vi "UHR-Fleezers Control (host) - 10.7.vi"() -> ()   [LabVIEW 2011] (continued)
  out "All Signals":waveform(dbl)[](graph)=[{"t0"=timestamp(6362.100000002397 s since 1904-01-01), "dt"=0.15, "Y"=[0.0, 0.0], "attributes"=variant("NI_ChannelName"=variant(string "APD 1"))}, {"t0"=timestamp(6362.100000002397 s since 1904-01-01), "dt"=0.15, "Y"=[0.0, 0.0], "attributes"=variant("NI_ChannelName"=variant(string "APD 2"))}, {"t0"=timestamp(6362.100000002397 s since 1904-01-01), "dt"=0.15, "Y"=[-0.08338581231742673, -0.0833608577290399], "attributes"=variant("NI_ChannelName"=variant(string "T1 Y"))}, {"t0"=timestamp(6362.100000002397 s since 1904-01-01), "dt"=0.15, "Y"=[-0.020466167643691944, -0.020695046740946327], "attributes"=variant("NI_ChannelName"=variant(string "T1 X"))}, {"t0"=timestamp(6362.100000002397 s since 1904-01-01), "dt"=0.15, "Y"=[0.05484865871150737, 0.05486028626361772], "attributes"=variant("NI_ChannelName"=variant(string "T1 Sum"))}, {"t0"=timestamp(6362.100000002397 s since 1904-01-01), "dt"=0.15, "Y"=[-0.08425842785872134, -0.08429414541514367], "attributes"=variant("NI_ChannelName"=variant(string "T2 Y"))}, {"t0"=timestamp(6362.100000002397 s since 1904-01-01), "dt"=0.15, "Y"=[-0.021052391190805018, -0.02125588256402392], "attributes"=variant("NI_ChannelName"=variant(string "T2 X"))}, {"t0"=timestamp(6362.100000002397 s since 1904-01-01), "dt"=0.15, "Y"=[0.054857295449689085, 0.05486660359507926], "attributes"=variant("NI_ChannelName"=variant(string "T2 Sum"))}, {"t0"=timestamp(6362.100000002397 s since 1904-01-01), "dt"=0.15, "Y"=[0.0185221741108709, 0.01777471038140605], "attributes"=variant("NI_ChannelName"=variant(string "T1 FB X"))}, {"t0"=timestamp(6362.100000002397 s since 1904-01-01), "dt"=0.15, "Y"=[0.007208807641834616, 0.007202642902920465], "attributes"=variant("NI_ChannelName"=variant(string "T1 FB Sum"))}, {"t0"=timestamp(6362.100000002397 s since 1904-01-01), "dt"=0.15, "Y"=[0.01339629623834087, 0.012486021324128876], "attributes"=variant("NI_ChannelName"=variant(string "T2 FB X"))}, {"t0"=timestamp(6362.100000002397 s since 1904-01-01), "dt"=0.15, "Y"=[0.007181218909268317, 0.007177312540055389], "attributes"=variant("NI_ChannelName"=variant(string "T2 FB Sum"))}, {"t0"=timestamp(6362.100000002397 s since 1904-01-01), "dt"=0.15, "Y"=[3.0154429223543846, 3.015887654048213], "attributes"=variant("NI_ChannelName"=variant(string "PSD Y"))}, {"t0"=timestamp(6362.100000002397 s since 1904-01-01), "dt"=0.15, "Y"=[0.1874808590976985, 0.18613934594687165], "attributes"=variant("NI_ChannelName"=variant(string "PSD X"))}, {"t0"=timestamp(6362.100000002397 s since 1904-01-01), "dt"=0.15, "Y"=[0.033047059541611565, 0.033048158207952705], "attributes"=variant("NI_ChannelName"=variant(string "PSD Y Sum"))}]
  in  "Signals to Plot":i32(listbox)
  out "Trap Disp. Freq. (Hz)":dbl=6.666666666666667 caption="Freq. (Hz)" format="%#_6p"
  out "Display Period (s)":dbl=0.15 caption="Period (s)" format="%#_6p"
  in  "Trap Disp. Downsample":dbl=10000.0 caption="Downsample" max=20000.0
  in  "APD Disp. Scale":dbl=0.1 caption="Scale (Divide,\nfor above plot only)"
  in  "APD Disp. Downsample":dbl=15.0 caption="Integrate" min=1.0 max=30.0 step=1.0
  out "APD Display Freq. (Hz)":dbl=6.666666666666667 caption="Freq. (Hz)"
  out "APD Display Period (s)":dbl=0.15 caption="Period (s)"
  out "FFT 1":cluster{"f0":dbl, "df":dbl, "magnitude":dbl[]}[](graph)=[{"f0"=0.0, "df"=3.3333333333333335, "magnitude"=array[10000 elements]}, {"f0"=0.0, "df"=3.3333333333333335, "magnitude"=array[10000 elements]}]
  out "FFT 2":cluster{"f0":dbl, "df":dbl, "magnitude":dbl[]}[](graph)
  in  "FFT 1 Choice 1":u16(ring) items=["T1 Y", "T1 X", "T1 Sum", "T2 Y", "T2 X", "T2 Sum", "T1 FB X", "T1 FB Sum", "T2 FB X", "T2 FB Sum", "PSD Y", "PSD X", "PSD Y Sum", "none"]
  in  "FFT 2 Choice 1":u16(ring)=13 items=["T1 Y", "T1 X", "T1 Sum", "T2 Y", "T2 X", "T2 Sum", "T1 FB X", "T1 FB Sum", "T2 FB X", "T2 FB Sum", "PSD Y", "PSD X", "PSD Y Sum", "none"]
  in  "FFT 1 Choice 2":u16(ring)=1 items=["T1 Y", "T1 X", "T1 Sum", "T2 Y", "T2 X", "T2 Sum", "T1 FB X", "T1 FB Sum", "T2 FB X", "T2 FB Sum", "PSD Y", "PSD X", "PSD Y Sum", "none"]
  in  "FFT 2 Choice 2":u16(ring)=13 items=["T1 Y", "T1 X", "T1 Sum", "T2 Y", "T2 X", "T2 Sum", "T1 FB X", "T1 FB Sum", "T2 FB X", "T2 FB Sum", "PSD Y", "PSD X", "PSD Y Sum", "none"]
  in  "Compute FFT":bool
  in  "Reset FFT":bool
  in  "# Spectra to Ave.":dbl=25.0
  out "Ave. Time (s)":dbl=7.5
  out "1 Channel":waveform(dbl)(graph)={"t0"=timestamp(0 s since 1904-01-01), "dt"=1.4999999999999999e-05, "Y"=array[20000 elements], "attributes"=variant("NI_ChannelName"=variant(string "T1 Y"))}
  out "Slow mean":dbl=-0.01200226252817839 format="%0.2f"
  in  "Slow mean N ave.":dbl=1.0 min=1.0 step=1.0
  out "Mean Intensity":dbl=-0.01200226252817839
  out "Sigma":dbl=0.006252248742901159
  out "Sigma/Mean":dbl=-0.5209225117532966
  in  "Subtract mean":bool
  in  "High Res. Display":u16(ring)=1 items=["T1 Y", "T1 X", "T1 Sum", "T2 Y", "T2 X", "T2 Sum", "T1 FB X", "T1 FB Sum", "T2 FB X", "T2 FB Sum", "PSD Y", "PSD X", "PSD Y Sum"]
  out "APD 1 Rate (Hz)":dbl format="%#_3p"
  in  "Tab Control":T4(tab)
  in  "11":bool
  out "Stage Moving":bool
  in  "Read Cal":bool
  in  "Confocal Linescan":bool
  in  "Speed (nm/s)":dbl=100.0
  in  "Furthest Withdraw (MHz)":dbl=15.0
  in  "Confocal Image":bool
  in  "Round T1 X":bool caption="Round"
  in  "T1 offset_x (mV)":dbl=24.980152760636827 format="%#_2g"
  in  "T1 kappa_x (pN/nm)":dbl=0.186857015570843 min=0.0 step=0.001 format="%#_2g"
  out "Total Time (s)":dbl=60.0
  in  "Start Saving":bool
  in  "Cal sets to save":u32=25 min=1 step=1
  in  "Comment (data description)":string="testing confocal setup"
  out "Calibrating Trap...":bool
  in  "Trap 2 (ON/OFF)":bool
  in  "Trap 1 (ON/OFF)":bool
  in  "Save Calibration":bool
  in  "N sets to save":u32=200 caption="N Sets"
  in  "Save N Sets":bool
  out "Save file name":path=path "E:/Data/111118/111118_038.dat"
  in  "Save ave N":dbl=250.0 caption="Averaging Factor"
  out "Saving...":bool
  in  "Stop Saving":bool
  out "Progress":u16(slide) scale=0.0..100.0
  out "Manipulating Trap":bool
  out "Buffer Status":dbl(slide) scale=0.0..1.0
  out "Overflow (data lost)":bool
  in  "Reset":bool
  out "Data Rate (Hz)":dbl=66666.66666666667 caption="Trap Data Rate (Hz)" format="%#_3p"
  out "Data Period (s)":dbl=1.4999999999999999e-05 caption="Trap Data Period (s)" format="%#_6p"
  out "Save Data Rate (Hz)":dbl=133.33333333333334 caption="Rate (Hz)" format="%#_6p"
  out "Save Data Period (s)":dbl=0.0075 caption="Period (s)" format="%#_6p"
  in  "T1 alpha_x (nm/V)":dbl=846.9258615688965 step=10.0 format="%#_3g"
  in  "T2 alpha_x (nm/V)":dbl=713.6162818729746 step=10.0 format="%#_3g"
  in  "T2 kappa_x (pN/nm)":dbl=0.23251742421714294 min=0.0 step=0.001 format="%#_2g"
  in  "T2 offset_x (mV)":dbl=21.883517478450205 format="%#_2g"
  in  "BD 1 Frequency 1 (MHz)":dbl=69.75 caption="T1 X (MHz)" min=60.0 max=90.0 step=1.0 format="%#_6p"
  in  "BD 1 Frequency 2 (MHz)":dbl=85.0 caption="T2 X (MHz)" min=60.0 max=90.0 step=1.0 format="%#_6p"
  in  "Green Laser ON/Interlacing":bool
  in  "Round T2 X":bool caption="Round"
  in  "AO1":dbl(slide)=6.552924588763087 caption="Confocal Y (V)" min=0.0 max=10.0 step=0.01 scale=0.0..10.0 scale format="%_1f"
  in  "AO2":dbl(slide)=1.456171758171331 caption="Confocal X (V)" min=0.0 max=10.0 step=0.01 scale=0.0..10.0 scale format="%_1f"
  in  "Trap Raster Scan":bool
  out "Raster Scanning...":bool
  in  "Trap Delta (MHz)":dbl=15.25
  in  "Setpoints (V)":cluster{"Set 1":dbl, "Set 2":dbl}={"Set 1"=9.0, "Set 2"=9.0}
  in  "Green FB Setpoint (mV)":dbl=90.0
  in  "Fish for Tether":bool
  in  "Position Label 5":string="upper flow spot (UvrD)" caption="5"
  in  "Move to Position":bool
  in  "Position":dbl=1.0 min=1.0 max=10.0 step=1.0
  in  "Set Position":bool
  in  "Saved Stage Positions":dbl[][](array[numeric])=[[1.0, 0.0, 0.0, 0.0], [2.0, -0.35449, -1.95512, -0.01509], [3.0, 1.5, -0.25, 0.0], [4.0, 0.1939, -2.16127, -0.03379], [5.0, 1.5, -2.0, -0.02], [6.0, 0.0, 0.0, 0.0], [7.0, 0.0, 0.0, 0.0], [8.0, 0.0, 0.0, 0.0], [9.0, 0.0, 0.0, 0.0], [10.0, 0.0, 0.0, 0.0]]
  in  "Move to Position 5":bool
  in  "z nudge increment (um)":dbl=0.5
  in  "+z":bool
  in  "Position 1 Label":string="Lower capillary (DNA beads)" caption="1"
  in  "Set Position 1":bool
  in  "Set Position 2":bool
  in  "Set Position 3":bool
  in  "Set Position 4":bool
  in  "Move to Position 3":bool
  in  "Move to Position 4":bool
  in  "Move to Position 2":bool
  in  "Move to Position 1":bool
  in  "Position 2 Label":string="Upper capillary (ADig beads)" caption="2"
  in  "Position 3 Label":string="lower flow spot (ATP)" caption="3"
  in  "Position 4 Label":string="Dump beads" caption="4"
  in  "-z":bool
  in  "Set Position 5":bool
  out "Stage Control Serial Error":errorcluster
  in  "Use Harvard pumps\nfor beads (else Chemyx)":bool=TRUE
  in  "Tab Control 9":enum32{"Harvard Pumps", "Chemyx Pumps"}(tab)
  out "P1 Flush Volume (uL)":dbl=183.5 caption="Volume (uL)"
  out "P3 Flush Volume (uL)":dbl=202.0 caption="Volume (uL)"
  out "P3 Flushing Bar":dbl(slide)=0.808 scale=0.0..1.0
  in  "Display On P3":bool caption="Display On"
  in  "Normal Flow Rate (ul/h) P3":dbl=400.0 caption="Normal Flow Rate (ul/h)"
  out "Flushing P3":bool caption="Flushing"
  in  "Retract Vol 1 (uL)":dbl=200.0 caption="Volume (uL)"
  in  "Retract Vol 3 (uL)":dbl=250.0 caption="Volume (uL)"
  in  "Retract Rate (uL/m)":dbl=2000.0
  in  "Retract Pump 1":bool
  in  "Retract Pump 3":bool
  in  "Stop Flow":bool
  in  "Start Flow":bool
  in  "Flush Sample":bool
  in  "Volume (uL)":dbl=75.0
  in  "Flush rate (uL/m)":dbl=100.0
  in  "Flow rate (uL/h)":dbl=100.0
  in  "Clear Volume":bool caption="Clear Infused Volume"
  in  "Flush Pump 3":bool
  in  "Volume (uL) P3":dbl=250.0 caption="Volume (uL)"
  in  "Flush rate (uL/m) P3":dbl=100.0 caption="Rate (uL/m)"
  out "Flushing P1":bool caption="Flushing"
  in  "Volume (uL) P1":dbl=200.0 caption="Volume (uL)"
  in  "Flush rate (uL/m) P1":dbl=100.0 caption="Rate (uL/m)"
  in  "Normal Flow Rate (ul/h) P1":dbl=800.0 caption="Normal Flow Rate (ul/h)"
  in  "Flush Pump 1":bool
  in  "Clear Volume P3":bool caption="Clear Infused Volume"
  in  "Clear Volume P1":bool caption="Clear Infused Volume"
  in  "Display On P1":bool caption="Display On"
  out "P1 Flushing Bar":dbl(slide)=0.9175 scale=0.0..1.0
  in  "All Pump Parameters":T5={"Pump 1"={"Diameter (mm)"=4.61, "Units"=4.0, "Volume"=100.0, "Rate"=25.0}, "Pump 2"={"Diameter (mm)"=4.61, "Units"=3.0, "Volume"=0.0, "Rate"=0.0}, "Pump 3"={"Diameter (mm)"=4.61, "Units"=4.0, "Volume"=100.0, "Rate"=800.0}}
  in  "Total Volume\nFlushed (uL)":dbl
  in  "Inject Pump 2":bool caption="Inject Pump 2\n(Flush Center)"
  in  "Flush Center Ch Rate (ul/m)":dbl=100.0
  in  "Flush Center Ch Volume (uL)":dbl=15.0
  in  "Pump pause delay (ms)":u32
  in  "Pump write delay (ms)":dbl=300.0
  in  "Ch 3 Inject Rate (ul/h)":dbl=800.0
  in  "Ch 3 Inject Volume (uL)":dbl=100.0
  in  "Ch 1 Inject Volume (uL)":dbl=100.0
  in  "Ch 1 Inject Rate (ul/h)":dbl=25.0
  out "Pump 1 cont disp":string="Right: DNA beads "
  out "Pump 3 cont disp":string="Left: ADig beads"
  in  "Read Harvard":bool
  out "read buffer":string
  out "Serial Settings:Number of Bytes at Serial Port":u32
  in  "write buffer":string
  in  "Tab Control 2":T6(tab)=enum."Feedback on Trap Position"
  out "Total Counts (ticks)":u32=600
  in  "Trap ON/OFF X or Y Amp?":bool=TRUE
  in  "Oscillate Set 1":bool
  in  "Trap 1 ON":bool
  in  "Number Interlace Sets":u8=3 min=1 max=3
  in  "DIO count 3 (ticks)":u32=200
  in  "DIO count 2 (ticks)":u32=200
  in  "DIO count 1 (ticks)":u32=200
  in  "BD 2 Amplitude 3 (%)":dbl min=0.0 max=50.0 step=1.0
  in  "BD 2 Amplitude 2 (%)":dbl min=0.0 max=50.0 step=1.0
  in  "BD 2 Amplitude 1 (%)":dbl min=0.0 max=50.0 step=1.0
  in  "BD 1 Amplitude 3 (%)":dbl min=0.0 max=50.0 step=1.0
  in  "BD 1 Amplitude 2 (%)":dbl=35.0 min=0.0 max=50.0 step=1.0
  in  "BD 1 Amplitude 1 (%)":dbl=10.0 min=0.0 max=50.0 step=1.0
  in  "BD 2 Frequency 3 (MHz)":dbl=26.0 min=0.0 max=40.0 step=1.0 format="%#_6p"
  in  "BD 1 Frequency 3 (MHz)":dbl=70.0 min=60.0 max=90.0 step=1.0 format="%#_6p"
  in  "BD 2 Frequency 2 (MHz)":dbl=26.0 min=0.0 max=40.0 step=1.0 format="%#_6p"
  in  "BD 2 Frequency 1 (MHz)":dbl=26.0 min=0.0 max=40.0 step=1.0 format="%#_6p"
  in  "Not-Interlacing Set":enum32{"Set 1", "Set 2", "Set 3"}(radio)
  in  "Interlace":bool=TRUE
  in  "Trap 2 ON":bool
  in  "Trap 3 ON":bool
  in  "Scan axis 2":bool=TRUE
  in  "Osc. freq. (Hz)":dbl=0.25
  in  "Osc. amp. (MHz)":dbl=2.0
  out "Coords":T7
  in  "Manipulation Scaling":cluster{"Horizontal":dbl, "Vertical":dbl}={"Horizontal"=0.075, "Vertical"=0.01}
  in  "Freq or Amp switch first":bool=TRUE
  in  "Swap F1 and F2":bool
  in  "Freq switch delay":u16
  in  "Amp switch delay":u16=5
  in  "MCL Step Increment (V_int)":dbl=3.0
  out "Time to Finish All (min)":dbl=0.13986 format="%#_2p"
  in  "Scan Speed (nm/s)":dbl=100.0
  in  "Scan Range (nm)":dbl=420.0
  in  "Step Size (nm)":dbl=1.0
  in  "MCL/AOM Scale Tweak":dbl=1.0
  in  "MCL Step Position Ratio":dbl=0.5
  in  "Move MCL Also?":bool=TRUE
  out "Final sep (nm)":dbl=1470.750000000001
  out "Initial sep (nm)":dbl=1050.75
  out "Save index":dbl=38.0
  out "Final delta (MHz)":dbl=18.66463414634147
  out "Initial delta (MHz)":dbl=15.25
  out "Final freq. (MHz)":dbl=66.33536585365853
  out "Initial freq. (MHz)":dbl=69.75
  in  "Saved AOD Raster Scan Parameter Sets":T8(array[cluster])=[{"Scan Range AOD (nm) 2"=500.0, "Step Size AOD (nm) 2"=1.0, "Scan Speed AOD (nm/s) 2"=100.0, "Number of scans (AOD) 2"=1, "Label"="offset curve"}, {"Scan Range AOD (nm) 2"=420.0, "Step Size AOD (nm) 2"=1.0, "Scan Speed AOD (nm/s) 2"=100.0, "Number of scans (AOD) 2"=1, "Label"="hp raster check"}, {"Scan Range AOD (nm) 2"=6.8, "Step Size AOD (nm) 2"=0.34, "Scan Speed AOD (nm/s) 2"=0.34, "Number of scans (AOD) 2"=1, "Label"="3.4 kbp - 1 bp steps"}, {"Scan Range AOD (nm) 2"=215.0, "Step Size AOD (nm) 2"=1.0, "Scan Speed AOD (nm/s) 2"=100.0, "Number of scans (AOD) 2"=3, "Label"="dt14 1 14 MHz start"}, {"Scan Range AOD (nm) 2"=450.0, "Step Size AOD (nm) 2"=1.0, "Scan Speed AOD (nm/s) 2"=100.0, "Number of scans (AOD) 2"=1, "Label"="dt14 2 small beads"}]
  in  "Load parameters":bool
  out "Scan Range (MHz)":dbl=-3.4146341463414633
  in  "Restart DMA? (AOD)":bool=TRUE caption="Restart DMA?"
  out "Incr. int (AOD)":i64=-7759651845
  out "Time/Scan (s) (AOD)":dbl=4.1958 format="%#_2p"
  out "Data points/scans":dbl=559440.0
  out "Data points/scan (f/b)":dbl=559440.0
  in  "Save scans":bool=TRUE
  out "AOD Scan I":u64=2 caption="Scan I"
  in  "Continuous AOD Scanning":bool caption="Continuous Scanning"
  in  "Abort AOD Scan":bool caption="Abort Scan"
  in  "Scan BD":bool=TRUE
  out "Cycles/step (AOD)":u64=666 format="%.3p"
  in  "Number of F/B Scans (AOD)":u16=1 min=1
  out "Scan steps (AOD)":u64=420
  out "Scan Increment (MHz)":dbl=-0.008149484836137144
  out "AOD Scanning":bool caption="Scanning"
  in  "Start AOD Scan":bool caption="Start Scan"
  out "N sets should be saved":dbl=27.972
  out "Progress 2":u16(slide) caption="Progress" scale=0.0..100.0
  in  "Abort save 2":bool caption="Abort save"
  in  "Trap 1 Bead Size (nm)":dbl=860.0
  in  "Trap 2 Bead Size (nm)":dbl=790.0
  out "MCL Count":dbl=782931.6080202643
  in  "All FB On/Off":bool=TRUE
  in  "AI2 to Setpoint":cluster{"Set 1":bool, "Set 2":bool}
  out "AI2 (V)":cluster{"Set 1":dbl, "Set 2":dbl}={"Set 1"=0.007019257179479354, "Set 2"=0.007019257179479354}
  in  "Reset Feedback":cluster{"Set 1":bool, "Set 2":bool}
  in  "PID Gains":T9={"Set 1"={"proportional gain (Kc)"=0, "integral gain (Kc*Ts/Ti)"=5, "derivative gain (Kc*Td/Ts)"=0}, "Set 2"={"proportional gain (Kc)"=0, "integral gain (Kc*Ts/Ti)"=5, "derivative gain (Kc*Td/Ts)"=0}}
  in  "Feedback On/Off":cluster{"Set 1":bool, "Set 2":bool}={"Set 1"=TRUE, "Set 2"=TRUE}
  in  "Rem fb disp offset":bool caption="Rem. Offset"
  in  "Remove Unwinding Offset":bool
  in  "FB Trap Pos Offset":dbl=-0.45359454723017834 caption="Offset (nm)" format="%.1f"
  in  "Negate Y Axis":bool=TRUE
  in  "Set Reading to\nSetpoint":bool
  out "Trap X (AI1)":T10={"Trap 1"=-0.2608642578125, "Trap 2"=-0.173919677734375}
  in  "Trap Pos FB SP":fxp<+/-,16,1>=-0.14154052734375 caption="Setpoint"
  in  "Trap Pos. FB ON":bool
  in  "Reset Trap Pos. FB":bool
  out "Trap Positions":waveform(dbl)[](graph)=[{"t0"=timestamp(6362.100000002397 s since 1904-01-01), "dt"=0.15, "Y"=[-0.45359454723017834, -0.45359454723017834], "attributes"=variant("NI_ChannelName"=variant(string "Trap 1 Pos."))}, {"t0"=timestamp(6362.100000002397 s since 1904-01-01), "dt"=0.15, "Y"=[-6.991740519879386e-12, -6.991740519879386e-12], "attributes"=variant("NI_ChannelName"=variant(string "Trap 2 Pos."))}]
  in  "Tab Control 8":enum32{"Main Setting", "Details"}(tab)=enum."Details"
  in  "Trap Pos FB Int Count":u16=100
  in  "Trap Pos. FB Gains":T11={"proportional gain (Kc)"=10.0, "integral gain (Kc*Ts/Ti)"=10.0, "derivative gain (Kc*Td/Ts)"=0.0} {"proportional gain (Kc)" format="%.11g"; "integral gain (Kc*Ts/Ti)" format="%.11g"; "derivative gain (Kc*Td/Ts)" format="%.11g"}
  in  "Negate Diff?":bool=TRUE
  in  "Differential FB?":bool=TRUE
  in  "Trap Pos. FB Offset Factor":i64=-440945501798
  in  "Trap Pos FB Negate Action":bool
  in  "Trap Pos. FB Mult Factor":i64=16777216
  in  "Trap Pos. AI1 X Pre-scale":u16
  in  "Trap Pos. FB Range":T12={"output high"=0.999969482421875, "output low"=-1.0}
  out "Trap Pos FB Int Signal":fxp<+/-,24,9>=-0.439361572265625 format="%.18g"
  out "Trap Pos FB Int-Norm Signal":fxp<+/-,16,1>=-0.00439453125 format="%.16g"
  in  "Set SP Using...":bool
  in  "Trap Pos FB Monitor\nT1 or T2":bool
  out "Trap X AI1 (DMA)":T13={"Set 1"=-0.02069091796875, "Set 2"=-0.021270751953125}
  in  "N El. to Ave.":dbl=10000.0
  out "Trap Pos FB Action":i64=-32768
  out "Action (%)":dbl(knob)=-100.0030518509476 scale=-100.0..100.0
  in  "Trap Pos. FB Out Scale 2^n":u8=24 caption="Action Scale Factor"
  out "Mean T1 Position (nm)":dbl=-0.45359454723017834 caption="Mean T1 (nm)" format="%0.2f"
  out "Trap 1 Position RMS (A)":dbl caption="RMS (Ang)"
  in  "Remove Action Offset":bool
  in  "factor":dbl=0.8
  in  "Trap Pos. Disp. Downsample":dbl=10000.0 caption="Trap Downsample"
  in  "Tab Control 3":enum32{"Timing", "MCL Scan", "Analog Out"}(tab)
  out "APD 2 Gate Late Counter":u32
  out "APD 2 Gate Relative Phase":i16
  in  "Phase Adj. (APD 2 Gate)":i16=20
  in  "Initial Phase Adjustment (APD 2 Gate)":i16=55
  out "APD 1 Gate Late Counter":u32
  in  "- phase (APD 1 Gate)":bool
  in  "+ phase (APD 1 Gate)":bool
  out "APD 1 Gate Relative Phase":i16
  in  "Phase Adj. (APD 1 Gate)":i16=20
  in  "Initial Phase Adjustment (APD 1 Gate)":i16=60
  in  "Save APD Data\nwith Trap Data":bool=TRUE
  out "APD FIFO Elements Remaining":u32
  in  "- phase (APD Acq)":bool
  in  "+ phase (APD Acq)":bool
  out "APD Acq Late Counter":u32
  out "APD Acq Relative Phase":i16
  in  "Phase Adj. (APD Acq)":i16=20
  in  "Initial Phase Adjustment (APD Acq)":i16
  in  "Invert APD Gate":bool caption="Invert Gate"
  in  "APD Gate OFF Count":u32=450 caption="Gate OFF Count"
  in  "APD Gate ON Count":u32=150 caption="Gate ON Count"
  in  "APD Gate":enum32{"ON", "OFF", "Interlace"}(radio)=enum."Interlace"
  in  "APD Integration Time (s)":dbl=0.01 caption="Integration Time (s)"
  out "APD Acq Rate (Hz)":dbl=100.0 caption="Rate (Hz)"
  out "APD Samples/FIFO Acq.":dbl=30.0
  out "APD Elements/DMA read":u32=60
  out "APD Int. Count":u32=400000 format="%.0p"
  in  "+ phase (APD 2 Gate)":bool
  in  "- phase (APD 2 Gate)":bool
  in  "Tab Control 5":enum32{"PSD X", "PSD Y", "Other Data Channel"}(tab)
  out "Data map":dbl[][](graph)=[[-0.04356808812995555, -0.043949990198051216, -0.04329247211298762, -0.044806914706250214, -0.04497006487399789, -0.045719005812832114, -0.04408359846885865, -0.04514353140221932, -0.041962582917125985, -0.04636550873593801, -0.043914619055159074, -0.04683532990207656, -0.04442546081662155, -0.04451819726481887, -0.042471011150113966, -0.04449502746456528, -0.04406110652401908, -0.04511356707532563, -0.043055846408805026, -0.04455325628948589], [-0.04272307183691837, -0.04298251116243269, -0.044576759741810634, -0.04463780503522186, -0.044225087510772865, -0.04443824322703492, -0.04337630149094779, -0.0453743121715329, -0.04418106930671227, -0.046052181179190965, -0.04300475075523317, -0.04553347975087725, -0.04359308720368342, -0.04490205649985289, -0.04397226744331681, -0.045061037321553796, -0.04287665703287454, -0.04402004381942739, -0.04279601151896481, -0.045509292947286784], [-0.04310481939323634, -0.0431361431679259, -0.04334195770022756, -0.0433235376897521, -0.04381115437785303, -0.043811554159733423, -0.043462557482984596, -0.04485439186110989, -0.043007740508463, -0.04494742195475332, -0.04406858632236289, -0.04553882519681925, -0.043894892940784795, -0.04449705033226854, -0.04284299378913778, -0.044579931435809086, -0.04359424536563487, -0.04489264824021985, -0.043332477526312294, -0.044896043605327465], [-0.0443705565670266, -0.04471294342428313, -0.04257750957517957, -0.043140526960799175, -0.04398459173658467, -0.0434113295488842, -0.04389803340354916, -0.042956598161319234, -0.0417056240208763, -0.0443941673878202, -0.043867927900175394, -0.0459520483406992, -0.0439523771011083, -0.04349943188909283, -0.042226825045218117, -0.04463076401444821, -0.04387236933422271, -0.04572330616817652, -0.0430271367534765, -0.04443744760566131], [-0.0430663909378329, -0.04650496765719157, -0.04407240998161559, -0.04494671869066438, -0.04295688856975709, -0.04114769967252234, -0.04208388990633566, -0.041016329828186225, -0.04197725061648673, -0.04268967245048369, -0.0420701342723601, -0.043167176464574165, -0.04298550876305195, -0.04402974602000453, -0.043451497500320735, -0.04459233086444822, -0.04278195684916027, -0.04443360960030157, -0.04275387512351318, -0.045588861147022236], [-0.04317822492916141, -0.04624126317678433, -0.04407187325142502, -0.04520108135653095, -0.04187270365564537, -0.04002822797530384, -0.04010201252531116, -0.03823218342638944, -0.039227537116352504, -0.038938173078962454, -0.03978030207117614, -0.04037402475500192, -0.04110689396684915, -0.04302816033357849, -0.04248193216247598, -0.0436215932332972, -0.04274547083843742, -0.0445518609027199, -0.042781429874380245, -0.04580593654981252], [-0.04469191631786788, -0.045143121001098935, -0.04142683255225041, -0.043352053215116634, -0.03985204309597411, -0.04031577561571997, -0.03827035809916074, -0.03504269720197355, -0.03462054591394463, -0.03490496605528337, -0.03702127192916683, -0.03774720087490985, -0.03886675034075545, -0.03915645595523903, -0.039969231620280446, -0.0424507149788552, -0.043151383051138525, -0.045109744688757225, -0.04319622028932636, -0.04450294735610162], [-0.044025199545637106, -0.04373367870378794, -0.04105064603430962, -0.041263723815150165, -0.03737517518972657, -0.03719982188864894, -0.03510921312023981, -0.03510865745233471, -0.033867221777986595, -0.033171020854609, -0.03463407124489765, -0.03365508017734025, -0.03637665754105138, -0.03690596379798225, -0.03935347391990818, -0.04134126023536294, -0.0421289690846951, -0.04371306985813796, -0.043282359855634764, -0.04515839144389473], [-0.04291394745892635, -0.04301145021196709, -0.04152463231414248, -0.039720914464388385, -0.03641474418961205, -0.0360487737234942, -0.0350464987444601, -0.03652448486346813, -0.03538378868256119, -0.036359728471222125, -0.034436686448390846, -0.03367456496549606, -0.03613765874241402, -0.0357703063449276, -0.0396435045983757, -0.04020270603864804, -0.041406256588181846, -0.04304303558205217, -0.043223007790289, -0.04555039102702618], [-0.043698951082245724, -0.042820923563118576, -0.039813513932712916, -0.039577697306068006, -0.03866744978408719, -0.039101331898438604, -0.03856514271690289, -0.03861949755426261, -0.03700785477107307, -0.03929574521155357, -0.03842125745453616, -0.04020088338493464, -0.03913379784646405, -0.036783575352205125, -0.03941734157301391, -0.03991548619712228, -0.043153250724085976, -0.04362114877356375, -0.04355756302746623, -0.04420345788543617], [-0.04379319504642183, -0.04273466735526933, -0.04160369439599057, -0.04179048263710069, -0.04194067709644228, -0.042114131831301256, -0.04174550007946842, -0.041580130189959166, -0.04116820580697224, -0.04308526196583359, -0.041841279633825175, -0.04448279050541758, -0.042865944528457274, -0.04202902489333639, -0.04217890164530165, -0.04170742315938955, -0.04417807762782673, -0.04296993598544083, -0.04481616066573546, -0.04372777751685604], [-0.04302232202984588, -0.043821993030143586, -0.04443399060267549, -0.04499853564120343, -0.044397543419309356, -0.04375482554944038, -0.044744940121372874, -0.04513587525816632, -0.046098241326348675, -0.04697850527511946, -0.04513771009928012, -0.04751660933759048, -0.04625986687095753, -0.04694561600622256, -0.04642565640023593, -0.04515334716318153, -0.0451955357781509, -0.04237372366638496, -0.04511732838834927, -0.04376032320273858], [-0.04424815920031558, -0.04482972156900288, -0.0452057348479569, -0.046273157790079344, -0.04777585017975011, -0.04781622248679544, -0.04855867678687889, -0.04848339351598763, -0.048809620738052326, -0.049586125157494124, -0.05003891320880427, -0.05083249422154624, -0.049589120738107936, -0.049795230657159385, -0.04789364477120554, -0.047798802267483426, -0.04722384757724611, -0.044367729774611384, -0.045184493997597996, -0.04276370236390873], [-0.04537394386185675, -0.04487468021340281, -0.04524829069036334, -0.047129242951336456, -0.04954091617586687, -0.05086315146113246, -0.051819030152760674, -0.05112555250950958, -0.05179024363657629, -0.05242672501390186, -0.05295302786747807, -0.05353303756731352, -0.05283148530526179, -0.049538659796130424, -0.048833637931339, -0.04788851721231732, -0.047215751290569624, -0.04744983826097653, -0.04356724561138798, -0.04283353387797738], [-0.04388485788863351, -0.04548089953352342, -0.046676466818111044, -0.04787032993825628, -0.04922298537808695, -0.05013447065845071, -0.052306917120640006, -0.053010292537097076, -0.05417203295290372, -0.05424471001747844, -0.05441214041597832, -0.05260569402390259, -0.05221508704942587, -0.049254833528896286, -0.049352809408869366, -0.04777287557485968, -0.044459808220892266, -0.045311253131667166, -0.042716418721233, -0.045360942370021154], [-0.04404439086464923, -0.04471221846091984, -0.04605178526157211, -0.046357764788920855, -0.0480862103185732, -0.049216325682016254, -0.05120514556444299, -0.05142738731325504, -0.05279106888159553, -0.05259783868498208, -0.05318487208781417, -0.05087788011188475, -0.05007098051412741, -0.047400036358575495, -0.04637185562052221, -0.045691133500629075, -0.042837863847997995, -0.045375029553818225, -0.042742504320083516, -0.0459312700955259], [-0.04544874326239919, -0.04398889751950914, -0.04441389974809712, -0.04444462228558817, -0.04630217962414502, -0.04822518330710934, -0.049331568369626516, -0.04767456957784551, -0.04969659341796623, -0.048905752418188335, -0.05070268292908432, -0.04939537604696824, -0.04701385639313278, -0.04437099431237157, -0.042574383421844025, -0.04435499850397863, -0.043452685342535075, -0.04558110997360502, -0.04404611668504134, -0.04445832830307417], [-0.04426407006696405, -0.044457111072996186, -0.04532574866538271, -0.04437385324271627, -0.04468867498432481, -0.04477113497355377, -0.047559630223499086, -0.046375185052936294, -0.04805650027584853, -0.04659404693085613, -0.04730877503050964, -0.04575934850278683, -0.04309864885105888, -0.04414288545233315, -0.04239599870606623, -0.043935226672855876, -0.04357940256802605, -0.04388183851877844, -0.04450265278601697, -0.044749086489306936], [-0.04440375314500626, -0.044749422903939545, -0.04549765882165978, -0.04496432796888508, -0.04531374625045316, -0.04326266460875787, -0.04642075469613538, -0.04502726046150156, -0.04717781940541915, -0.04613380869901115, -0.043768732180538825, -0.04468937769030085, -0.04235545914541923, -0.04368115387528518, -0.04349915605745644, -0.04385086373643782, -0.04366795248218799, -0.043743794660446304, -0.04459296017874259, -0.0449220320446585], [-0.045497640361173014, -0.043928922306644795, -0.04536539505075793, -0.043580675064850326, -0.04642775976943783, -0.044922155222188065, -0.04635567204934837, -0.04373138680598251, -0.04367264580732363, -0.044828230593413315, -0.04396253528092313, -0.0453430218854714, -0.043400786954471735, -0.042331216252329225, -0.04290959556255976, -0.043170550263441625, -0.04507765997676948, -0.04479329746312437, -0.044384731701121186, -0.04376196117274926], [-0.04630554626568874, -0.04427018638011891, -0.04622636104623591, -0.04349694278160117, -0.04608152384600206, -0.04398114355441808, -0.044060963858055135, -0.04392572843994412, -0.04323207428110669, -0.044867952468146594, -0.04425577149684179, -0.044993939478214076, -0.04461205396749994, -0.042697172664769384, -0.04351935096568463, -0.04347467355894634, -0.04483934609731635, -0.04414459348399515, -0.044713954437173464, -0.043792130924160795], [-0.046130924016695656, -0.04400096415516688, -0.04674642931595916, -0.04432808288055876, -0.0435445437017329, -0.0427258276772569, -0.04281011137952874, -0.04402524122503064, -0.044258699299539045, -0.045207767510811396, -0.04435047638218963, -0.04369948060778764, -0.04435555798251367, -0.043178045413062374, -0.044927126847892046, -0.04368420010888457, -0.04413712793755753, -0.04285930407916677, -0.04428921111174658, -0.044063906407558764], [-0.04663675523394236, -0.04410009599316418, -0.04478379254429056, -0.04328077396482595, -0.042828769143904884, -0.04392567964004893, -0.04351411076556656, -0.04325802413818074, -0.04414697242121593, -0.0441063153997706, -0.04562711680172417, -0.04405430935774726, -0.044598225231278335, -0.042284637407270134, -0.04407229266006496, -0.04299840255286558, -0.045198977363944105, -0.0440554281921161, -0.04429766079507033, -0.043100988216461605], [-0.04582325441515636, -0.04390471213348686, -0.04255365454157398, -0.04276547916511331, -0.0433035878387982, -0.04359875205512414, -0.044136487898170054, -0.04193534184922023, -0.043263043308499206, -0.042514719664123804, -0.04423064223732546, -0.04308192530049152, -0.044306378931007424, -0.04089100110258133, -0.04317806012610287, -0.04276220638057378, -0.04507940886963757, -0.044949516109338256, -0.04404033150355194, -0.04277041992588235], [-0.04262139158611726, -0.04405235896853276, -0.043431811178990316, -0.043689708761826485, -0.04311518785456257, -0.04058687051707326, -0.04273736607287319, -0.04063673343628279, -0.04251929789198451, -0.040869376698164636, -0.041662200984348474, -0.03970371947528775, -0.042131458375584005, -0.040406146132737165, -0.043621050490174604, -0.0423168423489198, -0.04330801074826586, -0.0432188627666502, -0.04411587280271885, -0.04392810211485355], [-0.042616412691845865, -0.04398772438364314, -0.043829021885562154, -0.04231479053665177, -0.04251711404278169, -0.03972359549073409, -0.04098331344346659, -0.03867063815404838, -0.04033317720508239, -0.038769320206477706, -0.0403955249978818, -0.038168611110994836, -0.04070112283877808, -0.038968732968358094, -0.041281636709806536, -0.04122762415894797, -0.04348467944423816, -0.04327830465463639, -0.043940175311722035, -0.043876291241745226], [-0.04285809598831744, -0.04342363835736864, -0.043170534740906784, -0.04077319574080924, -0.04161189461553155, -0.040142168670331865, -0.04090697388230026, -0.03722327311497742, -0.039971703792070504, -0.037656418861882826, -0.040323000468853384, -0.03906428977683192, -0.04033777796038948, -0.03738925514798844, -0.03992396150017499, -0.04027810149947197, -0.04368313499621269, -0.044071734781748195, -0.043424619343798126, -0.042554578160287154], [-0.04184906434687617, -0.04352997086691515, -0.04288196516137578, -0.041258357472587576, -0.0415514402650934, -0.038934422918446565, -0.04117466294942203, -0.03928544464099575, -0.04231580582374182, -0.040359553724815526, -0.04174223349816729, -0.03920891551071968, -0.0414084320630109, -0.03910832929397727, -0.041356502174967724, -0.040919933497661556, -0.04263962023732956, -0.042841711792952264, -0.04375937865298708, -0.04368710475120373], [-0.0422703512537065, -0.043706417337165876, -0.04298264593951273, -0.04267639872924073, -0.04230753546137646, -0.040366780226839205, -0.04311481215583279, -0.041479598600032655, -0.04452577971933616, -0.04278910405998204, -0.043608543520434785, -0.04120439247970654, -0.043246463301155835, -0.04136108088900986, -0.04297109885530703, -0.04167770238524134, -0.0429286644033242, -0.043049416617106574, -0.043764178625624706, -0.044037842901227725], [-0.04540655360874535, -0.04379321694788518, -0.04238262121563495, -0.04224062122146866, -0.04360541239751366, -0.04415331487874136, -0.04497660656323474, -0.043262072935799145, -0.045375254662329736, -0.0446059542140325, -0.04638339615613189, -0.04531622656688158, -0.04585228184924654, -0.04275826658694589, -0.043939216300324616, -0.042895455403780404, -0.045171552653411495, -0.044920705122636254, -0.044349837861881056, -0.042690879927039085], [-0.046381197905230195, -0.04424361331417134, -0.04481930665176647, -0.04372214809386149, -0.04411780764053787, -0.04510136506975617, -0.04519865549601501, -0.04578979664532344, -0.04705070158584583, -0.04732317001895543, -0.04811694599686227, -0.046958593970764406, -0.04747902832455568, -0.04572075680294631, -0.04594220667565587, -0.04440264753283646, -0.045971818506867615, -0.04453970322271603, -0.04474557365737013, -0.043223962422193535], [-0.04615124362383721, -0.04488164601028645, -0.047117310877995616, -0.04506952638110363, -0.045498821997111874, -0.04510810665386292, -0.04548023798096283, -0.04728986011983714, -0.04827745857907481, -0.04917635292372169, -0.04829919819341916, -0.04725149142378128, -0.04858257422317251, -0.04761635145578518, -0.04736595558632682, -0.04513489897698156, -0.04506436036000618, -0.04389384229385814, -0.04479788004639042, -0.044249790472432424], [-0.04631851526033104, -0.04468954022855416, -0.04602197366966188, -0.04430408931444463, -0.04747472999312401, -0.04681378460140095, -0.047215672483690754, -0.047386915127909074, -0.04693680058930991, -0.04900920333778939, -0.04829058695636229, -0.04906350762373441, -0.04860208155528013, -0.046733604457797936, -0.04533431371837946, -0.04448497157665671, -0.04583970934373692, -0.044812630392767006, -0.04526010338938975, -0.043562146591893836], [-0.04549527716560444, -0.04465046017461834, -0.045481774375945416, -0.043689016398658756, -0.04680344550979149, -0.04618476174876013, -0.04821887797431758, -0.04633559116830166, -0.04646881908021891, -0.04797592453683745, -0.047299919937968636, -0.04811903970223992, -0.046244394824051474, -0.045165462016064875, -0.044172737306834756, -0.04420653433858967, -0.04563239636258508, -0.04502970406168033, -0.04496273740265759, -0.043108137927933415], [-0.044524430546217665, -0.044243716543335546, -0.04542407587306845, -0.044437205502798435, -0.045664571481627184, -0.043909422456629245, -0.04639026774688232, -0.04546772161620838, -0.04782138614543838, -0.04728530595066164, -0.04498824140136454, -0.045036740720027904, -0.0438112901844491, -0.04533766915790395, -0.04368251711064636, -0.04422498873157607, -0.04412737209230293, -0.04339769939703596, -0.044918867287570635, -0.04426435851582551], [-0.044281024374307434, -0.044082163153445056, -0.04457500356298191, -0.04387962147036195, -0.04463836002371663, -0.04451585819534814, -0.04570280955753263, -0.044126070794909905, -0.04618395001957025, -0.04556983062086001, -0.046108699224811873, -0.04484104944800389, -0.043047095947796855, -0.04480225363474741, -0.042005610427670856, -0.04357733409678673, -0.04359369572087021, -0.04382126999504815, -0.04516857599655176, -0.044334658463518875], [-0.044988650081761596, -0.043770672856513856, -0.04339489236701542, -0.04336254671643143, -0.044367298208276826, -0.045773160791539313, -0.04493409666262693, -0.042743657009945514, -0.04491823409047242, -0.0447289691387146, -0.04646618441120952, -0.045867174909832886, -0.04494871685135195, -0.043831092762610914, -0.041120011166666415, -0.043228501509097725, -0.04345343898938096, -0.04527045325836227, -0.0436271281164915, -0.044108522212514566], [-0.04371934975462585, -0.04372664576142807, -0.04421555259715956, -0.044105549604542625, -0.04412356492123849, -0.04380822626169252, -0.04395392760545428, -0.04364689961449217, -0.045089771402014436, -0.04504004607204842, -0.04601648005902305, -0.044107646015539265, -0.045360795971124274, -0.04492863630249415, -0.044208238542553374, -0.043647904947070826, -0.04239012111715567, -0.044556946914350366, -0.04234693739489251, -0.045220053700609414], [-0.04337764569157828, -0.04383562034798598, -0.04407214924188177, -0.0437160699598084, -0.04333123212384861, -0.04321230748209906, -0.04375854421960602, -0.04375051779256926, -0.04470246087164729, -0.045430624327195024, -0.04548558755336504, -0.04412720029818729, -0.04588427971882829, -0.045185813799890125, -0.04560381017587637, -0.045068116809331704, -0.04369345908355131, -0.04467770263745831, -0.04196934492667104, -0.04515282224227886], [-0.04472049484462676, -0.04343411424228855, -0.04298593045807503, -0.04278723650167858, -0.04359398773951438, -0.04454687412629977, -0.044220727871246285, -0.04306223587169017, -0.04353295601255411, -0.04481714305018053, -0.04567586492421469, -0.04572859613952412, -0.046006245181920286, -0.04503809838029707, -0.044568511503901564, -0.04509940385717553, -0.04592749307275282, -0.04592467509025343, -0.042918112875085235, -0.042339740944127194]]
  in  "Channel":i32=4
  in  "Abort MCL Scan":bool
  out "MCL Scan I":u64=2
  out "MCL Scanning":bool
  in  "Start MCL Scan":bool
  out "wait to reset values":bool
  in  "Tab Control 4":enum32{"Scan Settings", "MCL FPGA Loop Timing"}(tab)
  out "Total Time (s)":dbl=48.0
  in  "Scan lines (y)":u64=20
  in  "Fast Scan Dir":bool=TRUE
  in  "2D or 1D Scan":bool=TRUE
  out "Initial X":dbl=-0.2763640247810297
  out "Initial Y":dbl=5.7432685323648816
  out "Time/f+b scan (s) (MCL)":dbl=2.4 caption="Time/scan (s)"
  in  "Number of scans (MCL)":u64=1 caption="Scans"
  in  "Scan steps (MCL)":u64=40 caption="Scan steps (x)"
  in  "N APD Samp/step":dbl=3.0
  in  "Scan Range (V)\n(of steps)":dbl=3.5
  in  "Restart DMA? (MCL)":bool=TRUE caption="Restart DMA?"
  in  "Continuous MCL Scanning":bool caption="Cont. Scanning"
  in  "Center Scan":bool=TRUE
  in  "Save Data (MCL)":bool=TRUE caption="Save Data"
  out "Actual Incr. int (MCL)":i16=294 caption="Incr. int"
  out "Desired incr (int)":dbl=294.0628205128205
  out "Desired Scan Incr (V)":dbl=0.08974358974358974
  out "N sets should be saved (MCL)":dbl=160.0 caption="N sets should be saved"
  out "Data points/scans (MCL)":dbl=4800.0 caption="Data points/scans"
  out "Data points/scan (f+b)":dbl=240.0 caption="points/scan (f+b)"
  out "Cycles/step (MCL)":u64=2000 caption="Cycles/step" format="%.0p"
  out "Actual MCL Inc (V)":dbl=0.08972441785943175
  in  "Phase adjust (MCL)":i16 caption="Phase adjust"
  out "Relative Phase (MCL)":i16 caption="Relative Phase"
  in  "Initial Phase Adj. (MCL)":i16 caption="Initial Phase Adj."
  in  "Update Count (MCL)":u32=600
  in  "+ phase (MCL)":bool
  in  "- phase (MCL)":bool
  out "MCL Late Counter":u32
  in  "APD 1 AO Mult.":i16=1 min=1
  in  "APD 2 AO Mult.":i16=1 min=1
  in  "Tab Control 7":enum32{"Green FB Signals", "Slow MCL Scan"}(tab)
  out "Green FB Plot":dbl(graph)=-0.010681478316599017
  out "MCL Scan 2":cluster{"Begin (V)":dbl, dbl, dbl[]}(graph)
  out "MCL Scan":cluster{"Begin (V)":dbl, dbl, dbl[]}(graph)
  in  "Green laser mode":enum32{"Laser ON", "Laser OFF", "Interlace"}(radio)=enum."Interlace"
  in  "GI Frequency, ON count":u32=150 min=1 step=1
  in  "Invert GI":bool
  out "GI Late Counter":u32
  in  "Phase adj. (GI)":i16=5
  out "GI relative phase":i16
  in  "+ phase (GI)":bool
  in  "Initial Phase Adjustment (GI)":i16=19
  in  "GI Frequency, OFF count":u32=450 min=1 step=1
  in  "- phase (GI)":bool
  out "Green FB Signals (V)":cluster{"Y":dbl, "X":dbl, "Sum":dbl}={"Y"=-936.2, "X"=-936.2, "Sum"=-0.010681478316599017}
  out "Relative phase (Green FB)":i16
  in  "+ phase (Green FB)":bool
  in  "- phase (Green FB)":bool
  out "Green FB Count":u32=600
  in  "Phase adj. (Green FB)":i16=10
  in  "Initial Phase Adjustment (Green FB)":i16=50
  in  "Green FB On/Off":bool=TRUE
  in  "Current When FB OFF (%)":dbl=87.0 min=0.0 max=100.0 step=1.0
  in  "Green int current ON count adj":u32=150
  in  "Green FB Gains":T14={"proportional gain (Kc)"=10, "integral gain (Kc*Ts/Ti)"=5, "derivative gain (Kc*Td/Ts)"=0}
  in  "- phase (GI) 2":bool
  in  "Initial Phase Adjustment (GI) 2":i16=-100
  in  "+ phase (GI) 2":bool
  out "GI relative phase 2":i16
  in  "Phase adj. (GI) 2":i16=20
  out "GI Late Counter 2":u32
  in  "On one out of X cycles":u32=1
  in  "Trap Position FIFO Depth":u32=300000 format="%.0p"
  in  "# Samples/trap":u32=20000 format="%.0p"
  out "Trap AI Elements/DMA read":u32=320000 format="%.0p"
  out "Ave. Rate (Hz)":dbl=200000.0 format="%#_6p"
  out "FIFO El. Rem.":u32 format="%.0p"
  in  "Phase adj. (AI1)":i16=15
  out "Relative phase (AI1)":i16
  in  "+ phase (AI1)":bool
  in  "- phase (AI1)":bool
  out "Late Counter (AI1)":u32
  in  "Initial Phase Adjustment (AI1)":i16=220
  out "AI rate (Hz)":dbl=200000.0 format="%#_6p"
  in  "AI Count (ticks)":u32=200
  out "# Samples/channel":u32=40000 format="%.0p"
  in  "Trap AI FIFO Depth":u32=600000 format="%.0p"
  in  "Detector Type":string(combo)="IR-QPD + PSD + FB-QPD X position"
  in  "N Acq Sets (Traps + Fl.)":i16=3
  in  "Sets to FIFO (Traps)":T15={"Set 1"=TRUE, "Set 2"=TRUE, "Set 3"=FALSE}
  in  "FPGA Ave.":dbl=1.0 min=1.0 step=1.0
  out "Ave. Period (s)":dbl=5e-06 format="%#_6p"
  out "DMA Update Period (s)":dbl=0.3
  out "FPGA Averaging":bool
  out "Trap Sets":u32=2
  out "Counts/DMA":dbl=12000000.0 format="%#_6p"
  out "Trap Pos FIFO El Remaining":u32=306
  out "Trap Pos Elements/DMA read":u32=120000 format="%.0p"
  out "Trap AI FIFO Timeout":u16
  out "Trap Pos FIFO Timeout":u16
  in  "Video Capture Rate (Hz)":dbl=30.0
  in  "Video Index":dbl=1.0 min=1.0 step=1.0
  in  "New Video File":bool
  in  "Save Video":bool
  in  "Reset Averaging":bool
  in  "Averaging":bool
  in  "Save Image":bool
  in  "Image Index":dbl=1.0 min=1.0
  out "Path Out":path
  in  "Center Point":cluster{"X":i32, "Y":i32}={"X"=335, "Y"=271}
  in  "Zoom Factor":sgl=7.0
  out "Window Size":cluster{"Width":i32, "Height":i32}
  out "Window Position":cluster{"X Position":i32, "Y Position":i32}={"X Position"=40, "Y Position"=40}
  in  "Initial Window Size":cluster{"Width":i32, "Height":i32}={"Width"=884, "Height"=619}
  in  "Initial Window Position":cluster{"X Position":i32, "Y Position":i32}={"X Position"=796, "Y Position"=4}
  in  "Intensity Upper":dbl=88.0
  in  "Intensity Lower":dbl=66.0
  out "error out":errorcluster
  out "error out 2":errorcluster
  in  "Bottom  1 Harvard Syringe Pump Serial Port":refnum<visa-resource-name>="Bottom1Harvard"
  in  "Center Harvard Syringe Pump Serial Port":refnum<visa-resource-name>="CenterHarvard"
  in  "Lost Tether Alarm Threshold (pN)":dbl=0.5
  in  "AOM X Cal (nm/MHz)":dbl=123.0
  in  "MCL X Cal (nm/V)":dbl=1070.0
  out "X RF Amplitude Limits (%)":T16={"Minimum"=0.0, "Maximum"=50.0, "Increment"=1.0}
  out "X RF Frequency Limits (MHz)":T16={"Minimum"=60.0, "Maximum"=90.0, "Increment"=1.0}
  out "Y RF Frequency Limits (MHz)":T16={"Minimum"=0.0, "Maximum"=40.0, "Increment"=1.0}
  out "Y RF Amplitude Limits (%)":T16={"Minimum"=0.0, "Maximum"=50.0, "Increment"=1.0}
  in  "Manip. X?":bool=TRUE
  in  "Manip. Y?":bool
  in  "Force Manip Abort":bool
  out "Read cal error":errorcluster
  in  "DAQ Delay (ms)":u32=1000
  in  "Start Scan":bool
  in  "Scan axis":bool=TRUE
  in  "Osc. amp. (V)":dbl=5.0
  in  "Osc. center (V)":dbl=5.0
  in  "Osc. freq. (Hz) 2":dbl=1.0
  in  "MCL Mode":u16(ring) items=["Manual Positioning", "Sinusoidal Wave", "Linear Scan"]
  in  "Begin (V)":dbl
  in  "End (V)":dbl=10.0
  in  "N Points":dbl=20.0
  in  "Delay to Interlace (s)":dbl
  in  "Delayed Interlace Start":bool
  in  "Read Lateness and Rel Phase":bool
  out "Vec Mean of T1 T2":dbl[](array[numeric])=[-0.033892434406208594, -0.03512047454126055]
  in  "Cal read wait (s)":u32=5
  out "Time tether formed":timestamp=timestamp(3404503973.340228 s since 1904-01-01)
  in  "Sample Chamber Stage Serial Port":refnum<visa-resource-name>="ASRL4::INSTR"
  in  "Chemyx Syringe Pump Serial Port":refnum<visa-resource-name>="ASRL3::INSTR"
  in  "Limit Min (MHz)":dbl=10.0 caption="Min (MHz)"
  in  "Limit Max (MHz)":dbl=16.0 caption="Max (MHz)"
  in  "Limits Enable":bool=TRUE caption="Enable"
  out "AI labels":string[](array[string])=["T1 Y", "T1 X", "T1 Sum", "T2 Y", "T2 X", "T2 Sum", "T1 FB X", "T1 FB Sum", "T2 FB X", "T2 FB Sum", "PSD Y", "PSD X", "PSD Y Sum"]
  in  "Save Trap Pos. Data":bool=TRUE
  in  "Lower Ch. Cap.":bool
  in  "Top 3 Harvard Syringe Pump Serial Port":refnum<visa-resource-name>="Top3Harvard"
  # "After"
  # "During"
  # "Trap On?"
  # "BD Flow ON?"
  # "Samp Flow ON?"
  # "Trap Trig. Fl.?"
  # "Zero It"
  # "Floor it\n(e.g., hp unwinding)"
  # "1"
  # "2"
  # "Trap Display:"
  # "APD Display:"
  # "DAQ"
  # "Trap Manipulation"
  # "Data Saving"
  # "Bead Calibration"
  # "Bottom Pump (#1)"
  # "Central Sample Channels"
  # "Top Pump (#3)"
  # "Rate param is ul/h\nVolume param is ul"
  # "Chemyx Pump 2"
  # "Units: \n1 = ml/m\n2 = ml/h\n3 = ul/m\n4 = ul/h"
  # "X"
  # "Y"
  # "Oscillate Set 1 freq. (debugging)"
  # "BD 1"
  # "BD 2"
  # "AOD Raster Scan"
  # "Approx. trap separations"
  # "X"
  # "Y"
  # "FPGA\nreading"
  # "DMA\ntransfer"
  # "APD Gates"
  # "APD 2"
  # "APD 1"
  # "X"
  # "2D"
  # "Y"
  # "1D"
  # "Green Laser Interlacing"
  # "Green FB Measurement"
  # "Digital Gate"
  # "Current Analog Control"
  # "Total AI Rates (NOT rates/trap)"
  # "(Samples/trap x Trap Sets)"
  # "(Samples/channel x\n8 if averaging (8 channels)\n4 if no averaging)"
  # "Trap 1"
  # "Trap 2"
  # "Flour./Trap 3"
  # "External Video Window"
  # "MCL Position Debugging"
  # "Temporary Control Storage\n(these used to be somewhere else, still want to keep them)"
  # "Y"
  # "X"
  # "Trap Position Difference Limits"
